vi "Save read.vi"(1 "Saveit cluster 1":T1, 2 "Load from backup":bool, 3 "Write":bool, 4 "Select File":u16(ring)=3 items=["MOT recapture", "Most recent expt", "Quadrupole trap", "MOT fill", "BEC", "FORT with transfers", "ZP beam align", "Test1", "Test2", "Align probe beam", "Test3", "Test4", "Test5", "Blank", "Roundtrip MOT recapture", "IP trap load recapture"]) -> (0 "Saveit cluster 2":T1)   [LabVIEW 2017]
doc: "This subVI save the Module List to a file, or alternatively reads in the Module List from a previously saved file. Dated backup files are saved simultaneously. Inputs are Write/Read, File name, Module List. Output is Module List, and done."
uses:
  globals/Modules global.vi
panel:
  out "date/time string":string="30_12_05"
  out "appended path":path=path "C:/Debbie/experiment stuff/B231/19 Experiment Control/Saved module lists/backups/Test5 Wed_ Dec 28_ 2005"
  out "Path":path=path "C:/Debbie/experiment stuff/B231/19 Experiment Control/Saved module lists/MOT fill"
  # "This subVI saves (or reads into) the Module List.  Dated backup files are saved simultaneously."
  # "Read"
  # "Enable  Time           Module                  Parameters (port)(line)   Comments                        which timing block"
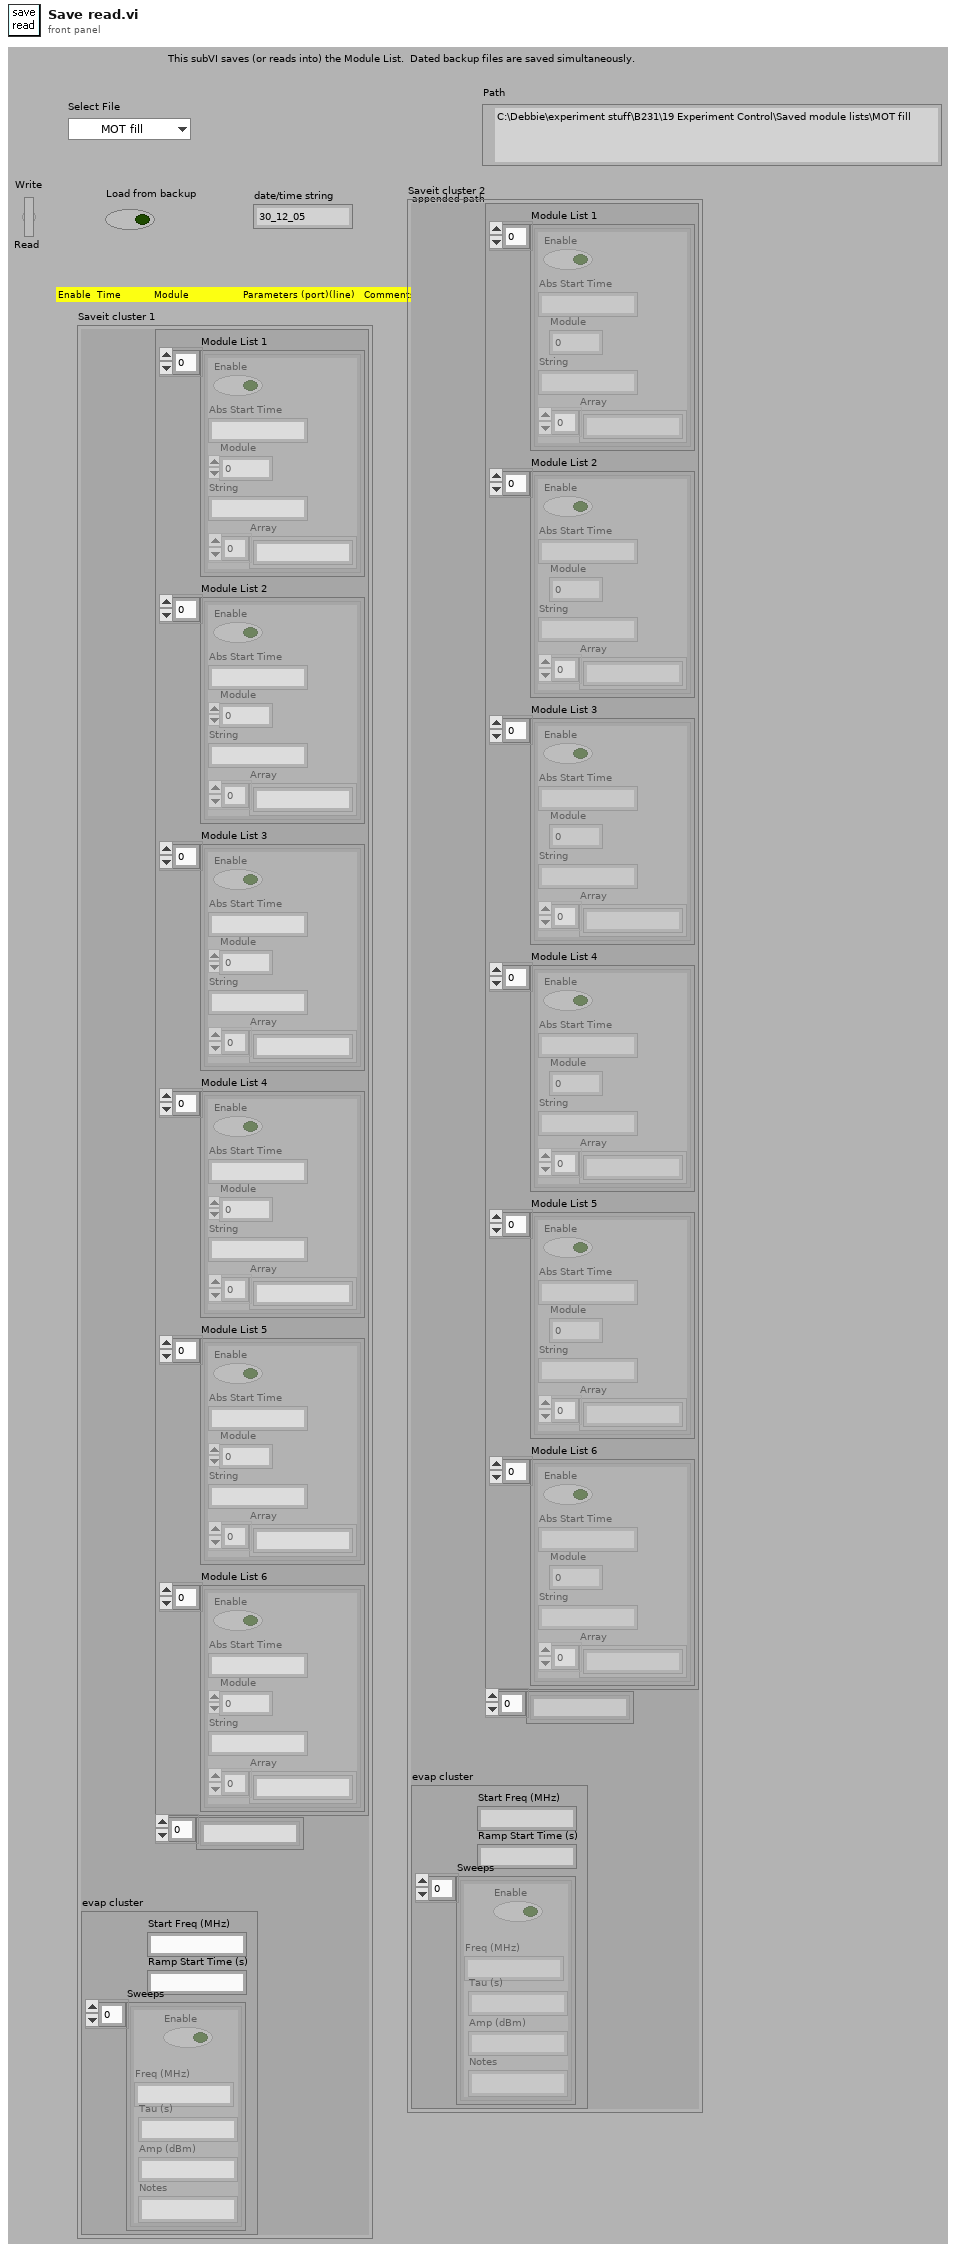
[diagram p1: front panel]
types:
  T1 = cluster{cluster{"Module List 1":cluster{"Enable":bool, "Abs Start Time":string, "Module":u16, "String":string, "Array":string[]}[], "Module List 2":cluster{"Enable":bool, "Abs Start Time":string, "Module":u16, "String":string, "Array":string[]}[], "Module List 3":cluster{"Enable":bool, "Abs Start Time":string, "Module":u16, "String":string, "Array":string[]}[], "Module List 4":cluster{"Enable":bool, "Abs Start Time":string, "Module":u16, "String":string, "Array":string[]}[], "Module List 5":cluster{"Enable":bool, "Abs Start Time":string, "Module":u16, "String":string, "Array":string[]}[], "Module List 6":cluster{"Enable":bool, "Abs Start Time":string, "Module":u16, "String":string, "Array":string[]}[]}, string[], "evap cluster":cluster{"Start Freq (MHz)":string, "Ramp Start Time (s)":string, "Sweeps":cluster{"Enable":bool, "Freq (MHz)":string, "Tau (s)":string, "Amp (dBm)":string, "Notes":string}[]}}
  T2 = enum16{"open", "replace", "create", "open or create", "replace or create", "replace or create with confirmation"}
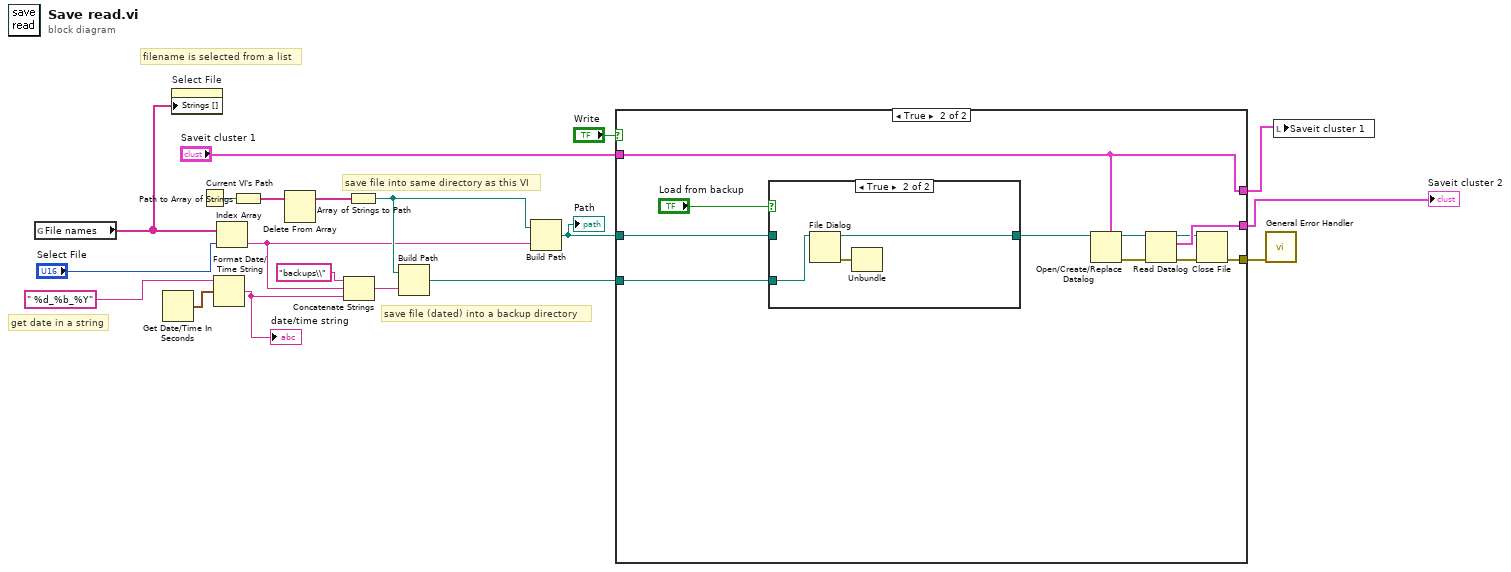
[diagram p0: block diagram]
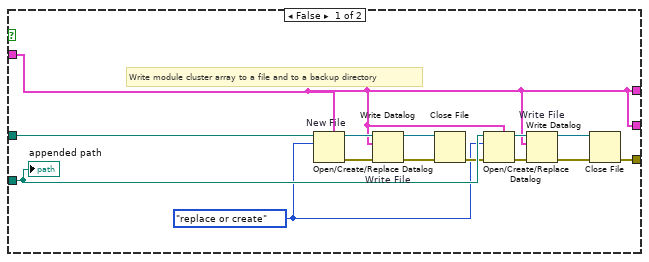
[diagram p2: hidden frame]
diagram:
  # "get date in a string"
  # "save file (dated) into a backup directory"
  # "save file into same directory as this VI"
  # "filename is selected from a list"
  n1 = global read "Modules global.vi" "File names"() -> (w12:string[])
  n2 = Get Date/Time In Seconds() -> (seconds since 1Jan1904=w11:timestamp)
  n3 = property on="Select File" class="Ring (strict)"("Strings []"=w12) -> ()  [unwired: 2 in, 2 out]
  n4 = Current VI's Path() -> (path=w19:path)
  n5 = Format Date/Time String(time format string (%c)=" %d_%b_%Y", seconds (now)=w11) -> (date/time string=w9:string)  [unwired: 1 in]
  "date/time string" <- w9
  n6 = Index Array(array=w12, index="Select File") -> (element=w8:string)
  n7 = Path to Array of Strings(0:w19) -> (2:w18:string[])  [unwired: 1 out]
  n8 = Delete From Array(array=w18) -> (array with subset deleted=w17:string[])  [unwired: 2 in, 1 out]
  n9 = Concatenate Strings("backups\\" ("Substring"), w8, w9) -> (w14:string)
  n10 = Array of Strings to Path(0:w17) -> (2:w15:path)  [unwired: 1 in]
  n11 = Build Path(base path=w15, name or relative path=w14) -> (appended path=w6:path)
  n12 = Build Path(base path=w15, name or relative path=w8) -> (appended path=w7:path)
  "Path" <- w7
  n13 = case shown="True" "Write" {
    tunnel: w7 -> [w22 w44]
    tunnel: w6 -> [w31 w41]
    tunnel: "Saveit cluster 1" -> [w21 w34]
    tunnel: [w24 w40] -> w4
    tunnel: [w21 w34] -> w2
    tunnel: [w21 w39] -> w1
    frame False {
      w20 = T2."replace or create" ("operation (0:open)")
      # "Write module cluster array to a file and to a backup directory"
      n14 = Open/Create/Replace Datalog "New File"(5:w21, 10:w20, 11:w22) -> (0:w27:errorcluster, 3:w32:refnum<k1>)  [unwired: 3 in, 1 out]
      n15 = Write Datalog "Write File"(4:w27, 6:w21, 7:w32) -> (0:w28:errorcluster, 3:w33:refnum<k1>)
      n16 = Close File(refnum=w33, error in=w28) -> (error out=w23:errorcluster)  [unwired: 1 out]
      n17 = Open/Create/Replace Datalog ("New File")(5:w21, 8:w23, 10:w20, 11:w31) -> (0:w25:errorcluster, 3:w29:refnum<k1>)  [unwired: 2 in, 1 out]
      n18 = Write Datalog "Write File"(4:w25, 6:w21, 7:w29) -> (0:w26:errorcluster, 3:w30:refnum<k1>)
      n19 = Close File(refnum=w30, error in=w26) -> (error out=w24:errorcluster)  [unwired: 1 out]
      "appended path" <- w31
    }
    frame True {
      n20 = case shown="True" "Load from backup" {
        tunnel: w44 -> [w45 _]
        tunnel: [w45 w48] -> w42
        tunnel: w41 -> [_ w47]
        frame False {
        }
        frame True {
          n21 = File Dialog(11:w47) -> (0:w46:errorcluster, 3:w48:path)  [unwired: 6 in, 2 out]
          n22 = Unbundle(w46) -> ()  [unwired: 3 out]
        }
      }
      n23 = Open/Create/Replace Datalog(5:w34, 11:w42) -> (0:w37:errorcluster, 3:w36:refnum<k1>)  [unwired: 4 in, 1 out]
      n24 = Read Datalog(4:w37, 7:w36) -> (0:w38:errorcluster, 2:w39:T1, 3:w35:refnum<k1>)  [unwired: 1 in]
      n25 = Close File(refnum=w35, error in=w38) -> (error out=w40:errorcluster)  [unwired: 1 out]
    }
  }
  "Saveit cluster 2" <- w1
  n26 = call <vilib>:"General Error Handler.vi"("error in (no error)"=w4) -> ()  [unwired: 10 in, 5 out]
  n27 = local write "Saveit cluster 1"(w2) -> ()
